vi "Close_Instr.vi"(8 "error in (no error)":errorcluster caption="entrée d'erreur (pas d'erreur)", 11 "Class Instrument Multimeter en entrée":refnum<class "Class Instrument Schielding_Box.lvclass">) -> (0 "error out":errorcluster caption="sortie d'erreur", 3 "Class Instrument Multimeter en sortie":refnum<class "Class Instrument Schielding_Box.lvclass">)   [LabVIEW 2020, in "Library Instrument & Equipement.lvlib" / "Library Instruments.lvlib" / "Class Instrument Schielding_Box.lvclass"]
uses:
  Class Instrument Schielding_Box.lvclass
  Class Instrument Schielding_Box.lvclass/Class Instrument Schielding_Box.ctl
  Shielding box/Class Shielding box (Default)/Class Shielding_ Box (Default).lvclass
  Instrument (Default)/Class Instrument (Default).lvclass
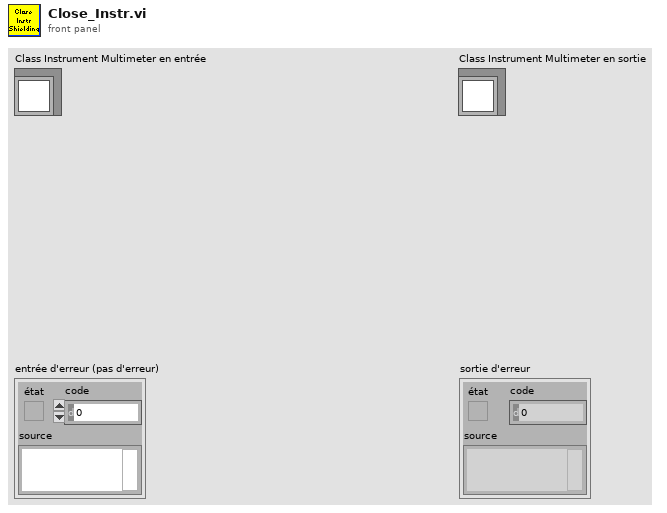
[diagram p1: front panel]
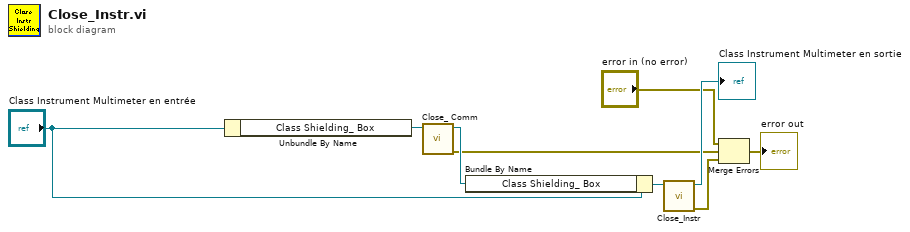
[diagram p0: block diagram]
diagram:
  n1 = Unbundle By Name("Class Instrument Multimeter en entrée") -> ("Class Shielding_ Box"=w3:refnum<class "Class Shielding_ Box (Default).lvclass">)
  n2 = call-dynamic "Close_ Comm.vi"("Class Shielding_ Box en entrée"=w3) -> ("error out"=w1:errorcluster, "Class Shielding_ Box en sortie"=w2:refnum<class "Class Shielding_ Box (Default).lvclass">)  [unwired: 9 in]
  n3 = Bundle By Name(cluster="Class Instrument Multimeter en entrée", "Class Shielding_ Box"=w2) -> (w7:refnum<class "Class Instrument Schielding_Box.lvclass">)
  n4 = call-parent "Close_Instr.vi"("Class Instrument (Default) en entrée"=w7) -> ("error out"=w5:errorcluster, "Class Instrument (Default) en sortie"=→"Class Instrument Multimeter en sortie":refnum<class "Class Instrument Schielding_Box.lvclass">)  [unwired: 9 in]
  n5 = Merge Errors("error in (no error)", w1, w5) -> (→"error out":errorcluster)
